vi "Initialize Hardware.vi"(8 "error in (no error)":errorcluster, 10 "Instruments":refnum<class "Instrument.lvclass">[](array[class]), 11 "Application in":refnum<class "Application.lvclass">) -> (0 "error out":errorcluster, 3 "Application out":refnum<class "Application.lvclass">)   [LabVIEW 2017, in "Application.lvlib" / "Application.lvclass"]
uses:
  Application.lvclass
  Instruments/Instrument/Class/Instrument.lvclass
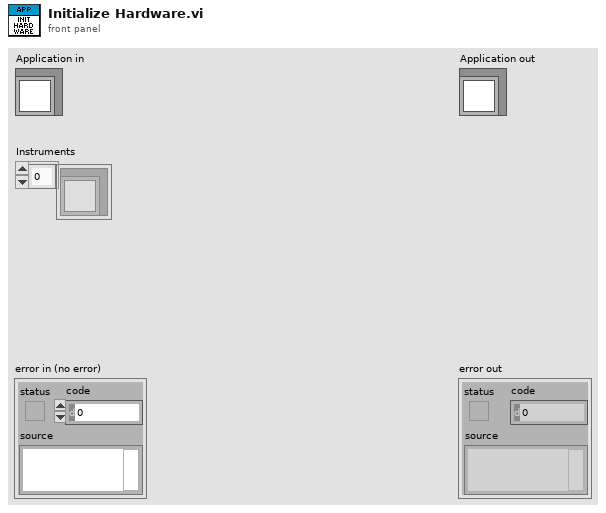
[diagram p1: front panel]
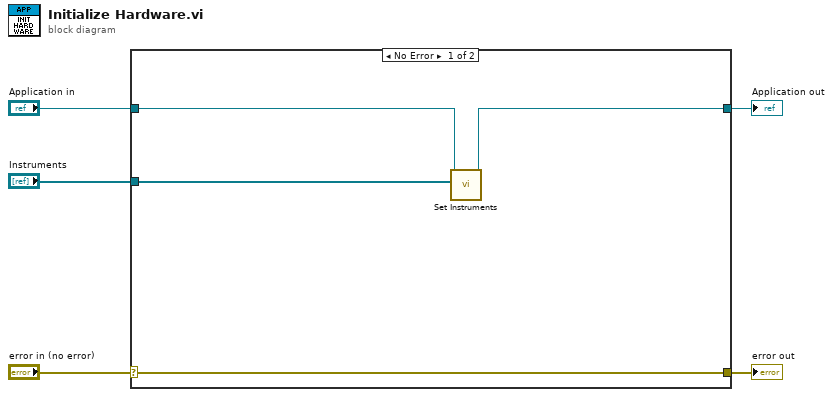
[diagram p0: block diagram]
diagram:
  n1 = case shown="No Error" "error in (no error)" {
    selector: "error in (no error)" -> [w9 w11]
    tunnel: [w9 w11] -> w4
    tunnel: [w7 w10] -> w2
    tunnel: "Application in" -> [w8 w10]
    tunnel: "Instruments" -> [w6 _]
    frame No Error {
      n2 = call "Set Instruments.vi"("Instruments"=w6, "Acrobat Template in"=w8) -> ("Acrobat Template out"=w7:refnum<class "Application.lvclass">)  [unwired: 8 in, 1 out]
    }
    frame Error {
    }
  }
  "error out" <- w4
  "Application out" <- w2
